vi "Open VI Reference.vi"(8 "error in (no error)":errorcluster, 11 "method":string) -> (0 "error out":errorcluster, 3 "VI out":refnum<vi>)   [LabVIEW 2016]
uses:
  Classes/Server/JSONRPC Server.lvclass
  Classes/Request/Request.lvclass
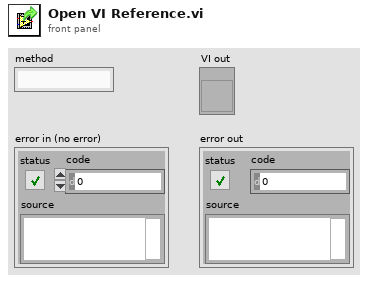
[diagram p1: front panel]
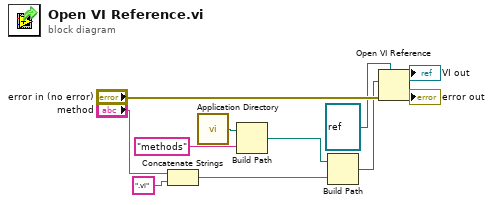
[diagram p0: block diagram]
diagram:
  n1 = Concatenate Strings("method", ".vi" ("string")) -> (w4:string)
  n2 = call <vilib>:"Application Directory.vi"() -> ("Application Directory"=w1:path)
  n3 = Build Path(base path=w1, name or relative path="methods") -> (appended path=w3:path)
  n4 = Build Path(base path=w3, name or relative path=w4) -> (appended path=w7:path)
  n5 = Open VI Reference(type specifier VI Refnum (for type only)=refnum<vi> refnum, vi path=w7, error in (no error)="error in (no error)") -> (vi reference=→"VI out":refnum<vi>, error out=→"error out":errorcluster)  [unwired: 3 in]
